vi "XML_EndMessage.vi"(10 "TestFixtureNumber":string, 11 "TestProgramVersion":string) -> (3 "连接的字符串":string)   [LabVIEW 2018]
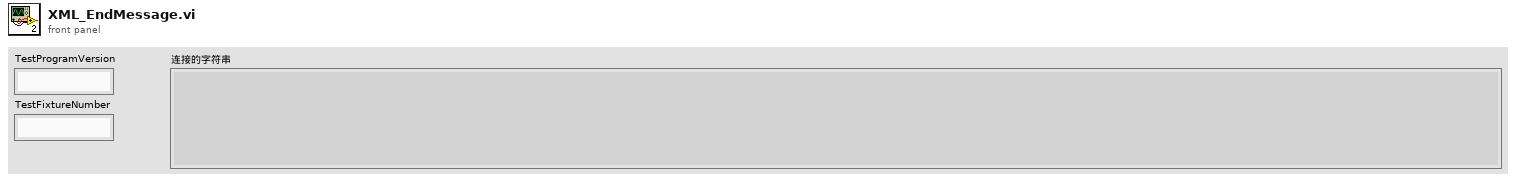
[diagram p1: front panel]
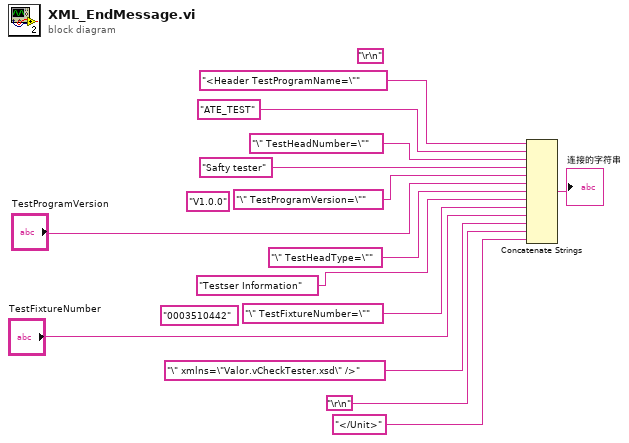
[diagram p0: block diagram]
diagram:
  (unwired) "0003510442"
  (unwired) "V1.0.0"
  (unwired) "\r\n"
  n1 = Concatenate Strings("<Header TestProgramName=\"", "ATE_TEST", "\" TestHeadNumber=\"", "Safty tester", "\" TestProgramVersion=\"", "TestProgramVersion", "\" TestHeadType=\"", "Testser Information", "\" TestFixtureNumber=\"", "TestFixtureNumber", "\" xmlns=\"Valor.vCheckTester.xsd\" />", "\r\n", "</Unit>") -> (→"连接的字符串":string)
